vi "write_practice.vi"() -> ()   [LabVIEW 2011]
uses:
  <vilib>/Utility/miscctls.llb/LVDateTimeRec.ctl
panel:
  out "date time rec":T1
  in  "file path (use dialog)":path
  out "output cluster":cluster{i32, "number: 0 to 1":dbl}
  out "Waveform Chart":dbl(graph)
  in  "millisecond multiple":u32
  out "number (0 to 1)":dbl
  in  "stop":bool
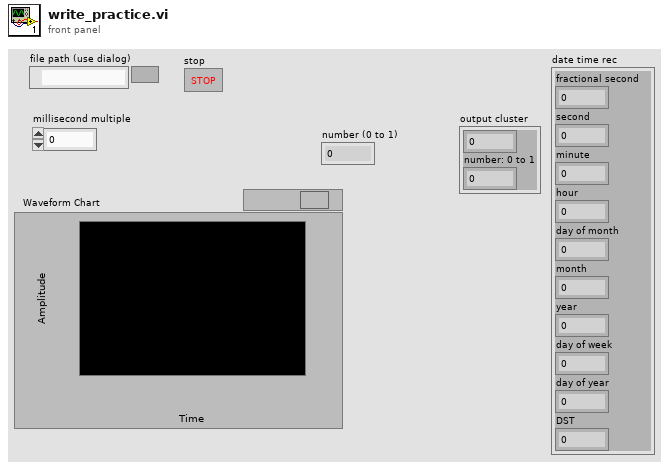
[diagram p1: front panel]
types:
  T1 = typedef "LVDateTimeRec.ctl" = cluster{"fractional second":dbl, "second":i32, "minute":i32, "hour":i32, "day of month":i32, "month":i32, "year":i32, "day of week":i32, "day of year":i32, "DST":i32}
  T2 = enum16{"open", "replace", "create", "open or create", "replace or create", "replace or create with confirmation"}
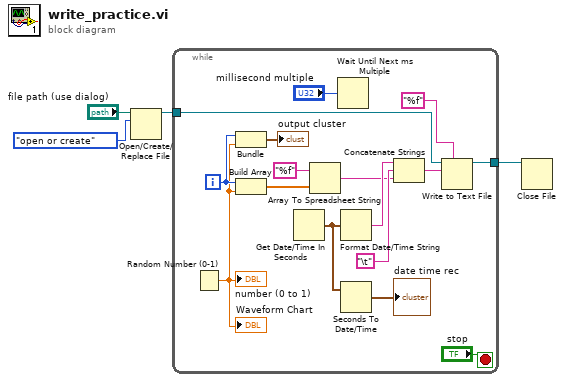
[diagram p0: block diagram]
diagram:
  n1 = Open/Create/Replace File(file path (use dialog)="file path (use dialog)", operation (0:open)=T2."open or create") -> (refnum out=w3:refnum<file>)  [unwired: 4 in, 2 out]
  n2 = while {
    tunnel: w3 -> [w15]
    tunnel: [w14] -> w2
    i -> [w13]
    stop <- "stop" stop-if-true
    n3 = Random Number (0-1)() -> (number: 0 to 1=w12:dbl)
    "number (0 to 1)" <- w12
    "Waveform Chart" <- w12
    n4 = Bundle(w13, "number: 0 to 1"=w12) -> (→"output cluster":cluster{i32, "number: 0 to 1":dbl})  [unwired: 1 in]
    n5 = Build Array(w13, w12) -> (w11:dbl[])
    n6 = Get Date/Time In Seconds() -> (seconds since 1Jan1904=w18:timestamp)
    n7 = Array To Spreadsheet String(array=w11, 3:"%f" ("format string")) -> (spreadsheet string=w5:string)  [unwired: 1 in]
    n8 = Wait Until Next ms Multiple(millisecond multiple="millisecond multiple") -> ()  [unwired: 1 out]
    n9 = Format Date/Time String(seconds (now)=w18) -> (date/time string=w6:string)  [unwired: 2 in]
    n10 = Seconds To Date/Time(time stamp (now)=w18) -> (date time rec=→"date time rec":T1)  [unwired: 1 in]
    n11 = Concatenate Strings(w6, "\t", w5) -> (w9:string)
    n12 = Write to Text File(prompt (Choose or enter file path)="%f", file (use dialog)=w15, text=w9) -> (refnum out=w14:refnum<file>)  [unwired: 1 in, 2 out]
  }
  n13 = Close File(refnum=w2) -> ()  [unwired: 1 in, 2 out]
